vi "超标留样启动流程.vi"   [LabVIEW 2016, in "超标留样集成.lvlib" / "ESTD1200.lvlib"]
uses:
  ESTD1200.lvlib
types:
  T1 = typedef "队列data.ctl" = cluster{"命令":string, "data":cluster{"站号":u16, "控制命令":u16[]}}
  T2 = cluster{"命令":string, "data":cluster{"站号":u16, "控制命令":u16[]}}
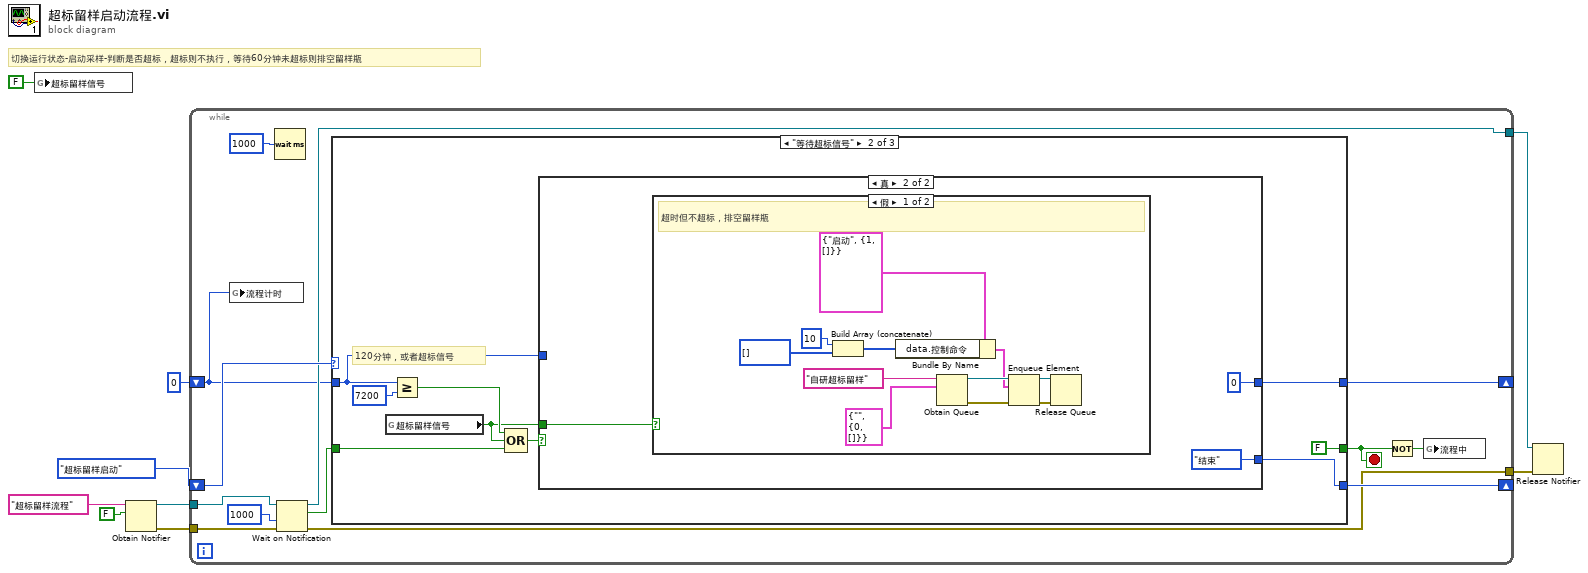
[diagram p0: block diagram]
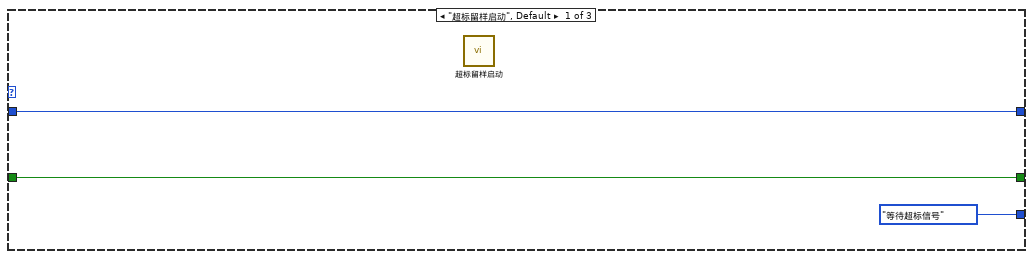
[diagram p2: hidden frame]
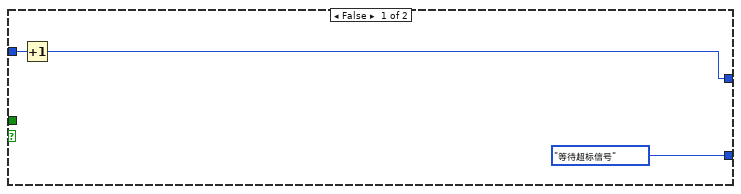
[diagram p3: hidden frame]
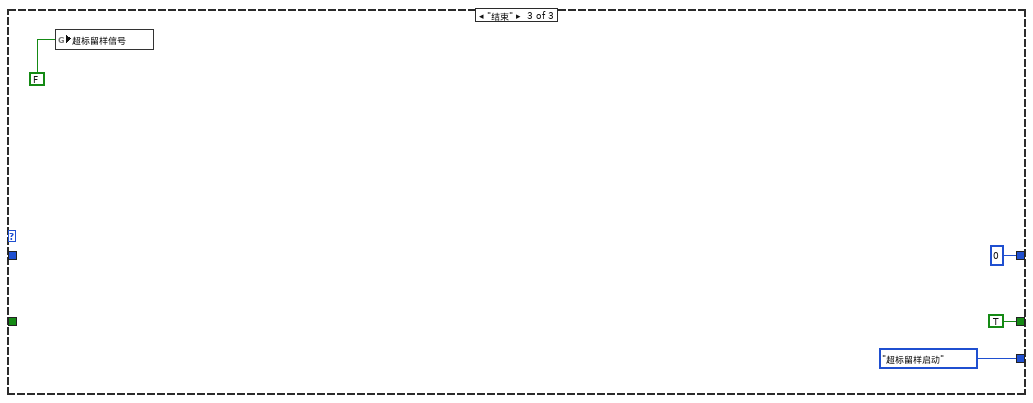
[diagram p5: hidden frame]
diagram:
  # "切换运行状态-启动采样-判断是否超标，超标则不执行，等待60分钟未超标则排空留样瓶"
  n1 = global write "串口参数断电保存全局变量.vi" "超标留样信号"(FALSE ("采样完成")) -> ()
  n2 = Obtain Notifier(name (unnamed)="超标留样流程" ("名称（未命名）"), notification data type=FALSE ("采样完成")) -> (notifier out=w5:refnum<notifier>, error out=w4:errorcluster)  [unwired: 2 in, 1 out]
  n3 = while {
    shift-right: [w16] -> _
    shift-left: enum16{"超标留样启动", "等待超标信号", "结束"}."超标留样启动" -> [w22]
    shift-right: [w20] -> _
    shift-left: 0 -> [w10]
    tunnel: w5 -> [w19]
    tunnel: w4 -> [w18]
    tunnel: [w12] -> w2
    tunnel: [w11] -> w1
    stop <- w13 stop-if-true
    n4 = global write "串口参数断电保存全局变量.vi" "流程计时"(w10) -> ()
    n5 = Wait (ms)(milliseconds to wait=u32 1000 ("等待时间（毫秒）")) -> ()  [unwired: 1 out]
    n6 = Wait on Notification(notifier=w19, timeout in ms (-1)=1000 ("超时毫秒(-1)"), error in (no error)=w18) -> (notifier out=w12:refnum<notifier>, notification=w14:bool, error out=w11:errorcluster)  [unwired: 1 in, 1 out]
    n7 = case shown="\"等待超标信号\"" w22 {
      tunnel: w10 -> [w24 w30 _]
      tunnel: [w24 w32 0] -> w20
      tunnel: [enum16{"超标留样启动", "等待超标信号", "结束"}."等待超标信号" w29 enum16{"超标留样启动", "等待超标信号", "结束"}."超标留样启动"] -> w16
      tunnel: [w23 FALSE TRUE] -> w13
      tunnel: w14 -> [w23 w26 _]
      frame "超标留样启动", Default {
        n8 = call "超标留样启动.vi"() -> ()  [unwired: 11 in, 1 out]
      }
      frame "等待超标信号" {
        # "120分钟，或者超标信号"
        n9 = global read "串口参数断电保存全局变量.vi" "超标留样信号"() -> (w27:bool)
        n10 = Greater Or Equal?(x=w30, y=7200) -> (x >= y?=w33:bool)
        n11 = Compound Arithmetic op=OR ("复合运算")(w33, w27, w26) -> (w31:bool)
        n12 = case shown="真" w31 {
          tunnel: [enum16{"超标留样启动", "等待超标信号", "结束"}."等待超标信号" enum16{"超标留样启动", "等待超标信号", "结束"}."结束"] -> w29
          tunnel: w30 -> [w37 _]
          tunnel: [w36 0] -> w32
          tunnel: w27 -> [_ w38]
          frame False {
            n13 = Increment(x=w37) -> (x+1=w36:i32)
          }
          frame True {
            n14 = case shown="假" w38 {
              frame False {
                # "超时但不超标，排空留样瓶"
                n15 = Build Array (concatenate)(u16 10 ("数值"), u16[] [] ("控制命令")) -> (w43:u16[])
                n16 = Bundle By Name(cluster=T2 {"命令"="启动", "data"={"站号"=1, "控制命令"=[]}} ("元素"), "data.控制命令"=w43) -> (w42:T2)
                n17 = Obtain Queue(name (unnamed)="自研超标留样" ("名称（未命名）"), element data type=T1 {"命令"="", "data"={"站号"=0, "控制命令"=[]}}) -> (queue out=w48:refnum<queue>, error out=w49:errorcluster)  [unwired: 3 in, 1 out]
                n18 = Enqueue Element(queue=w48, element=w42, error in (no error)=w49) -> (queue out=w50:refnum<queue>, error out=w51:errorcluster)  [unwired: 1 in, 1 out]
                n19 = Release Queue(queue=w50, error in (no error)=w51) -> ()  [unwired: 1 in, 3 out]
              }
              frame True {
                # "超标留样"
              }
            }
          }
        }
      }
      frame "结束" {
        n20 = global write "串口参数断电保存全局变量.vi" "超标留样信号"(FALSE ("采样完成")) -> ()
      }
    }
    n21 = Not(x=w13) -> (.not. x?=w15:bool)
    n22 = global write "串口参数断电保存全局变量.vi" "流程中"(w15) -> ()
  }
  n23 = Release Notifier(notifier=w2, error in (no error)=w1) -> ()  [unwired: 1 in, 3 out]
